vi "DC Centered Spectrum.vi"() -> ()   [LabVIEW 2023]
doc: "This VI demonstrates how to convert a signal to a standard DC centered spectrum by using the Nyquist shift modulation by alternating +1 and -1."
uses:
  <vilib>/Analysis/2dsp.llb/Power Spectrum (DBL).vi
  <vilib>/Analysis/0measdsp.llb/Scaled Time Domain Window (DBL).vi
  <vilib>/Analysis/NI_AALPro.lvlib
  <vilib>/Analysis/NI_AALBase.lvlib
panel:
  in  "Window":u32(ring) items=["Rectangle"=0, "Hanning"=1, "Hamming"=2, "Blackman-Harris"=3, "Exact Blackman"=4, "Blackman"=5, "Flat Top"=6, "4 Term B-Harris "=7, "7 Term B-Harris"=8, "Low Sidelobe"=9, "Blackman Nuttall"=11, "Triangle"=30, "Bartlett-Hanning"=31, "Bohman"=32, "Parzen"=33, "Welch"=34, "Kaiser"=60, "Dolph-Chebyshev"=61, "Gaussian"=62]
  in  "Apply Window":bool=TRUE
  out "Waveform Signal":dbl[](graph)
  out "Noise Signal":dbl[](graph)
  in  "Noise Type Distribution":u16(ring)=2 items=["Gaussian", "Rectangular", "Periodic", "Bernoulli", "Poison"]
  in  "Signal":u16(ring) items=["Sine", "Square", "Triangle", "Sawtooth", "Arbitrary", "Swept Sine"]
  in  "Noise Level":dbl(slide)=0.1 scale=0.0..1.0
  in  "Stop":bool
  in  "Frequency (Hz)":dbl(slide)=100.0 scale=1.0..200.0
  out "Modulated Signal to Shift Spectrum":dbl[](graph)
  out "DC-Centered Power Spectrum":cluster{i32, dbl, "Power Spectrum":dbl[]}(graph)={-256, 1.0, "Power Spectrum"=[]}
  # "Description: Demonstrates how to convert a signal to a standard DC centered power spectrum through modulation.\nRequirements: LabVIEW Full Development System\nInstructions:\n1. Run the VI.  Change the Frequency. You can add noise by selecting the Noise Type Distribution and increasing the Noise Level. \n2. View the DC-Centered Power Spectrum, which shows the spectrum of the signal after it is modulated by alternating +1 and -1 (Nyquist frequency).\n3. Click Stop to stop the VI."
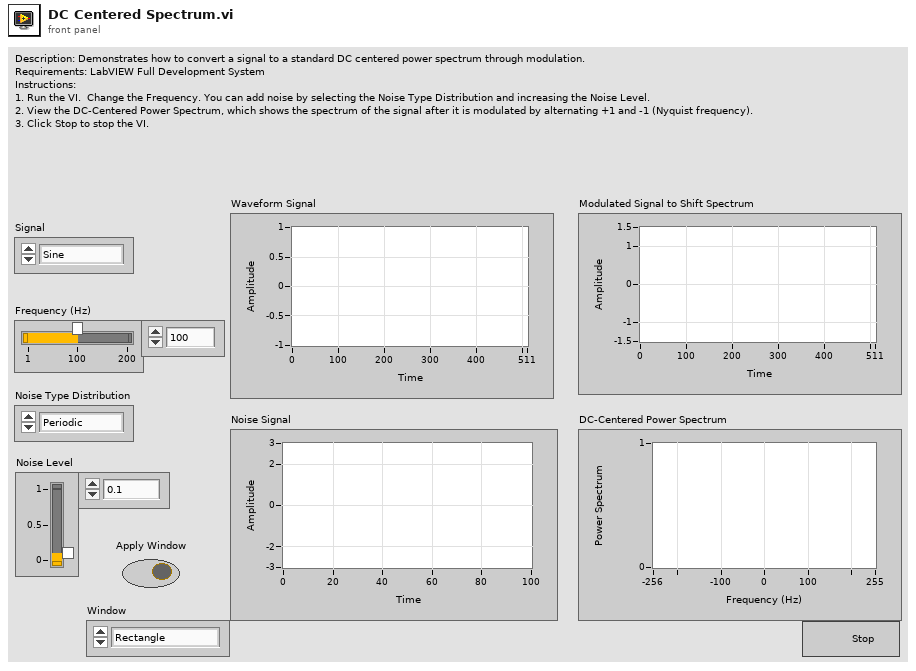
[diagram p1: front panel]
types:
  T1 = cluster{"Number of samples":i32, dbl, "Power Spectrum":dbl[]}
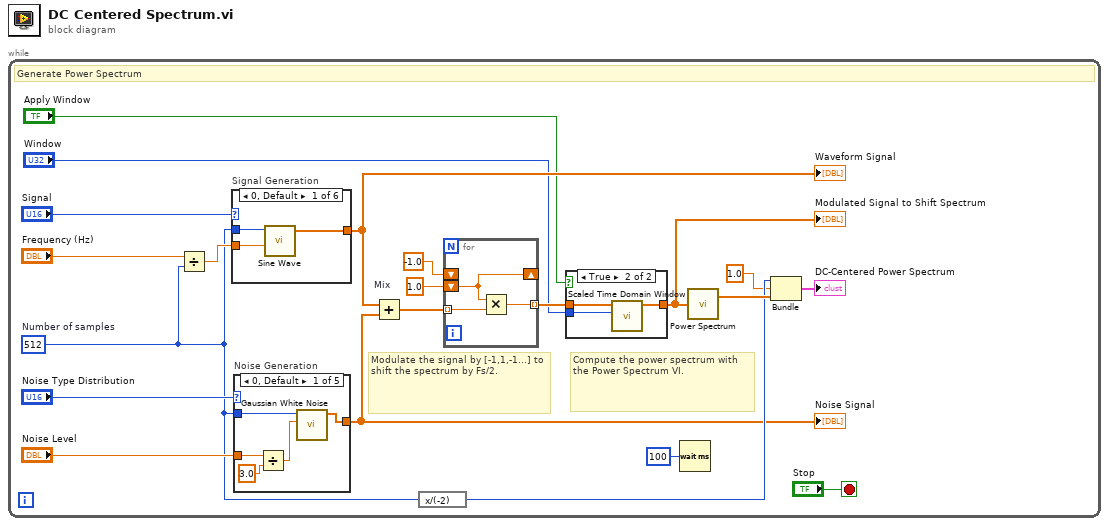
[diagram p0: block diagram]
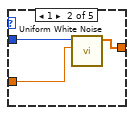
[diagram p3: hidden frame]
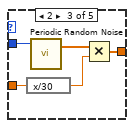
[diagram p4: hidden frame]
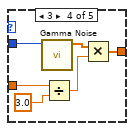
[diagram p5: hidden frame]
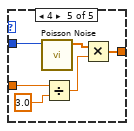
[diagram p6: hidden frame]
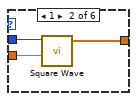
[diagram p7: hidden frame]
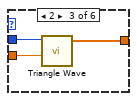
[diagram p8: hidden frame]
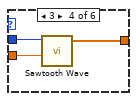
[diagram p9: hidden frame]
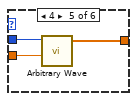
[diagram p10: hidden frame]
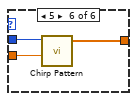
[diagram p11: hidden frame]
diagram:
  n1 = while {
    stop <- "Stop" stop-if-true
    w2 = 512  # Number of samples
    # "Compute the power spectrum with the Power Spectrum VI."
    # "Modulate the signal by [-1,1,-1...] to shift the spectrum by Fs/2."
    # "Generate Power Spectrum"
    n2 = Divide(x="Frequency (Hz)", y=w2) -> (x/y=w13:dbl)
    n3 = case "Signal Generation" shown="0, Default" "Signal" {
      tunnel: [w56 w59 w62 w65 w68 w71] -> w10
      tunnel: w2 -> [w55 w58 w61 w64 w67 w70]
      tunnel: w13 -> [w54 w57 w60 w63 w66 w69]
      frame 0, Default {
        n4 = call <vilib>:"Sine Wave.vi"("samples"=w55, "frequency"=w54) -> ("sine wave"=w56:dbl[])  [unwired: 3 in, 2 out]
      }
      frame 1 {
        n5 = call <vilib>:"Square Wave.vi"("samples"=w58, "frequency"=w57) -> ("square wave"=w59:dbl[])  [unwired: 4 in, 2 out]
      }
      frame 2 {
        n6 = call <vilib>:"Triangle Wave.vi"("samples"=w61, "frequency"=w60) -> ("triangle wave"=w62:dbl[])  [unwired: 3 in, 2 out]
      }
      frame 3 {
        n7 = call <vilib>:"Sawtooth Wave.vi"("samples"=w64, "frequency"=w63) -> ("sawtooth wave"=w65:dbl[])  [unwired: 3 in, 2 out]
      }
      frame 4 {
        n8 = call <vilib>:"Arbitrary Wave.vi"("frequency"=w66, "samples"=w67) -> ("arbitrary wave"=w68:dbl[])  [unwired: 5 in, 2 out]
      }
      frame 5 {
        n9 = call <vilib>:"Chirp Pattern.vi"("f1"=w69, "samples"=w70) -> ("Chirp Pattern"=w71:dbl[])  [unwired: 2 in, 1 out]
      }
    }
    "Waveform Signal" <- w10
    n10 = case "Noise Generation" shown="0, Default" "Noise Type Distribution" {
      tunnel: [w33 w36 w39 w45 w51] -> w11
      tunnel: "Noise Level" -> [w32 w35 w38 w44 w50]
      tunnel: w2 -> [w31 w34 w40 w46 w52]
      frame 0, Default {
        n11 = Divide(x=w32, y=3.0 ("x")) -> (x/y=w30:dbl)
        n12 = call <vilib>:"Gaussian White Noise.vi"("standard deviation"=w30, "samples"=w31) -> ("Gaussian noise pattern"=w33:dbl[])  [unwired: 8 in, 1 out]
      }
      frame 1 {
        n13 = call <vilib>:"Uniform White Noise.vi"("amplitude"=w35, "samples"=w34) -> ("uniform white noise"=w36:dbl[])  [unwired: 8 in, 1 out]
      }
      frame 2 {
        n14 = expression code="x/30"(w38) -> (w37:dbl)
        n15 = call <vilib>:"Periodic Random Noise.vi"("samples"=w40) -> ("periodic random noise"=w41:dbl[])  [unwired: 2 in, 1 out]
        n16 = Multiply(x=w41, y=w37) -> (x*y=w39:dbl[])
      }
      frame 3 {
        n17 = call <vilib>:"Gamma Noise.vi"("samples"=w46) -> ("gamma noise"=w47:dbl[])  [unwired: 9 in, 1 out]
        n18 = Divide(x=w44, y=3.0 ("x")) -> (x/y=w43:dbl)
        n19 = Multiply(x=w47, y=w43) -> (x*y=w45:dbl[])
      }
      frame 4 {
        n20 = call <vilib>:"Poisson Noise.vi"("samples"=w52) -> ("poisson noise"=w53:dbl[])  [unwired: 9 in, 1 out]
        n21 = Divide(x=w50, y=3.0) -> (x/y=w49:dbl)
        n22 = Multiply(x=w53, y=w49) -> (x*y=w51:dbl[])
      }
    }
    "Noise Signal" <- w11
    n23 = Add "Mix"(x=w10, y=w11) -> (x+y=w9:dbl[])
    n24 = expression code="x/(-2)"(w2) -> (w19:i32)
    n25 = for {
      shift-right: [w26] -> _
      shift-left: -1.0 -> [_]
      shift-left: 1.0 -> [w26]
      tunnel: w9 -> [w28] mode=indexing
      tunnel: [w27] -> w8 mode=indexing
      n26 = Multiply(x=w26, y=w28) -> (x*y=w27:dbl)
    }
    n27 = case shown="True" "Apply Window" {
      tunnel: w8 -> [w22 w25]
      tunnel: [w22 w24] -> w6
      tunnel: "Window" -> [_ w23]
      frame False {
      }
      frame True {
        n28 = call-poly <vilib>:"Scaled Time Domain Window.vi"("window"=w23, "X"=w25) -> ("Windowed X"=w24:dbl[])  [unwired: 7 in, 2 out]
      }
    }
    "Modulated Signal to Shift Spectrum" <- w6
    n29 = Wait (ms)(milliseconds to wait=u32 100 ("millisecond multiple")) -> ()  [unwired: 1 out]
    n30 = call-poly <vilib>:"Power Spectrum.vi"("X"=w6) -> ("Power Spectrum"=w21:dbl[])  [unwired: 1 out]
    n31 = Bundle("Number of samples"=w19, 1.0, "Power Spectrum"=w21) -> (→"DC-Centered Power Spectrum":T1)  [unwired: 1 in]
  }
